vi "Continuous Pulse Train Test (audio).vi"() -> ()   [LabVIEW 2015]
uses:
  Waveform VIs/Pulse Train VIs/Pulse Train Params.ctl
  Waveform VIs/Pulse Train VIs/Pulse Polarity.ctl
  Waveform VIs/Pulse Train VIs/PT-Continuous State.ctl
  <vilib>/sound2/lvsound2.llb/Sound Data Format.ctl
  <vilib>/sound2/lvsound2.llb/Sampling Mode.ctl
  <vilib>/sound2/lvsound2.llb/Sound Output Write (DBL Single).vi
panel:
  in  "Phase (cycles)":dbl(slide)=1.0 min=0.0 max=1.0 scale=0.0..1.0
  in  "stop":bool
  in  "Sound Format":T1={"sample rate (S/s)"=50000.0, "number of channels"=2, "bits per sample"=16}
  in  "Device ID":u32
  in  "Pulse Train Params":T2={"Pulse width (us)"=100.0, "Pulse rate (Hz)"=0.0, "Gap (ms)"=0.0, "Polarity"=enum."NEG-POS", "PT State"={"Template"=[], "Nperiod"=0, "Index"=0, "Pulse Rate (Hz)"=0.0, "Phase (cycles)"=0.0, "Noff"=0}, "Asynch"=FALSE}
  out "Graph":dbl[](graph)
  in  "Buffer (ms)":dbl=100.0
  in  "Pulse Rate (Hz)":dbl(slide)=36.55555555555556 min=1.0 max=100.0 scale=1.0..100.0
  in  "Fs (Hz)":dbl=100000.0
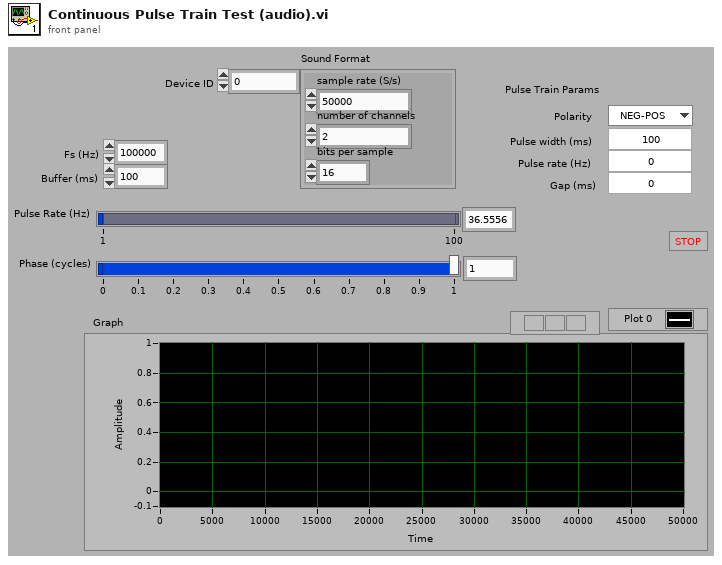
[diagram p1: front panel]
types:
  T1 = typedef "Sound Data Format.ctl" = cluster{"sample rate (S/s)":dbl, "number of channels":i32, "bits per sample":i32}
  T2 = typedef "Pulse Train Params.ctl" = cluster{"Pulse width (us)":dbl, "Pulse rate (Hz)":dbl, "Gap (ms)":dbl, "Polarity":T3, "PT State":T4, "Asynch":bool}
  T3 = typedef "Pulse Polarity.ctl" = enum16{"POS", "NEG", "POS-NEG", "NEG-POS"}
  T4 = typedef "PT-Continuous State.ctl" = cluster{"Template":dbl[], "Nperiod":i32, "Index":i32, "Pulse Rate (Hz)":dbl, "Phase (cycles)":dbl, "Noff":i32}
  T5 = typedef "Sampling Mode.ctl" = i32
  T6 = typedef "Sound Output Task ID.ctl" = u32
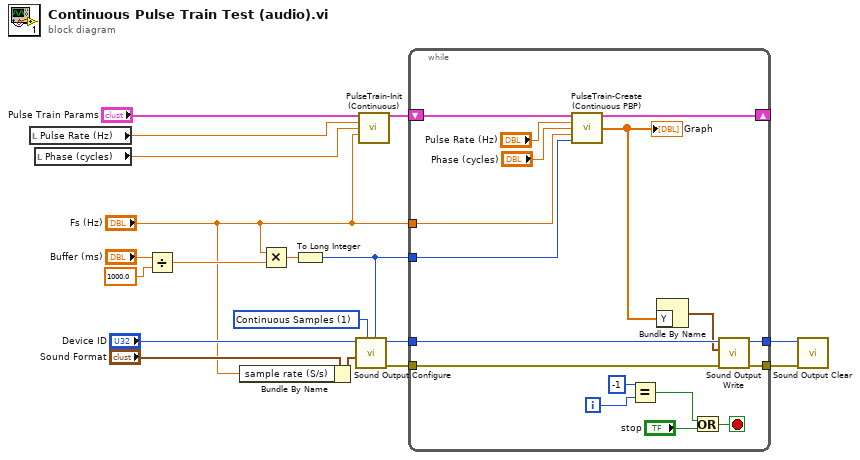
[diagram p0: block diagram]
diagram:
  w11 = T5 1 items=["Finite Samples", "Continuous Samples"] ("sample mode")
  n1 = local read "Pulse Rate (Hz)"() -> (w2:dbl)
  n2 = local read "Phase (cycles)"() -> (w1:dbl)
  n3 = Divide(x="Buffer (ms)", y=1000.0) -> (x/y=w16:dbl)
  n4 = Bundle By Name(cluster="Sound Format", "sample rate (S/s)"="Fs (Hz)") -> (w9:T1)
  n5 = Multiply(x="Fs (Hz)", y=w16) -> (x*y=w15:dbl)
  n6 = To Long Integer(number=w15) -> (32bit integer=w8:i32)
  n7 = call <vilib>:"Sound Output Configure.vi"("number of samples/ch"=w8, "sample mode"=w11, "sound format"=w9, "device ID"="Device ID") -> ("error out"=w5:errorcluster, "task ID"=w6:T6)  [unwired: 6 in]
  n8 = call "PulseTrain-Init (Continuous).vi"("Pulse Train Params"="Pulse Train Params", "Start Pulse Rate (Hz)"=w2, "Start Phase (cycles)"=w1, "Fs (Hz)"="Fs (Hz)") -> ("Initial State"=w14:T4)  [unwired: 10 in, 1 out]
  n9 = while {
    tunnel: w8 -> [w26]
    tunnel: "Fs (Hz)" -> [w25]
    shift-right: [w34] -> _
    shift-left: w14 -> [w35]
    tunnel: w6 -> [w31]
    tunnel: w5 -> [w32]
    tunnel: [w30] -> w4
    tunnel: [w29] -> w3
    i -> [w21]
    stop <- w23 stop-if-true
    n10 = call "PulseTrain-Create (Continuous PBP).vi"("State In"=w35, "Pulse Rate (Hz)"="Pulse Rate (Hz)", "Phase (cycles)"="Phase (cycles)", "Fs (Hz)"=w25, "Npts"=w26) -> ("State Out"=w34:T4, "Buffer"=w19:dbl[])  [unwired: 8 in, 1 out]
    "Graph" <- w19
    n11 = Equal?(x=-1, y=w21) -> (x = y?=w20:bool)
    n12 = Bundle By Name("Y"=w19) -> (w27:waveform(dbl))  [unwired: 1 in]
    n13 = Or(x=w20, y="stop") -> (x .or. y?=w23:bool)
    n14 = call-poly <vilib>:"Sound Output Write.vi"("error in (no error)"=w32, "data"=w27, "task ID"=w31) -> ("error out"=w29:errorcluster, "task ID out"=w30:T6)  [unwired: 7 in]
  }
  n15 = call <vilib>:"Sound Output Clear.vi"("error in (no error)"=w3, "task ID"=w4) -> ()  [unwired: 9 in, 1 out]
